vi "步骤树形列表（子VI）.vi"(5 "数据数组":string[][](array[string]), 6 "数据存储时间间隔（分钟）":dbl format="%#g", 7 "停止":bool, 8 "error out":errorcluster, 9 "queue out":refnum<queue>, 10 "数组":string[][](array[string]), 11 "notifier out":refnum<notifier>) -> (0 "当前步骤":i32, 1 "多位阀的位置":string)   [LabVIEW 2016]
uses:
  <vilib>/Utility/file.llb/Write Delimited Spreadsheet (string).vi
panel:
  out "跳转次数变量":i32=2
  out "报警器":i32
  out "电磁阀2":i32
  out "电磁阀1":i32
  out "气泵":i32
  out "蠕动泵":i32
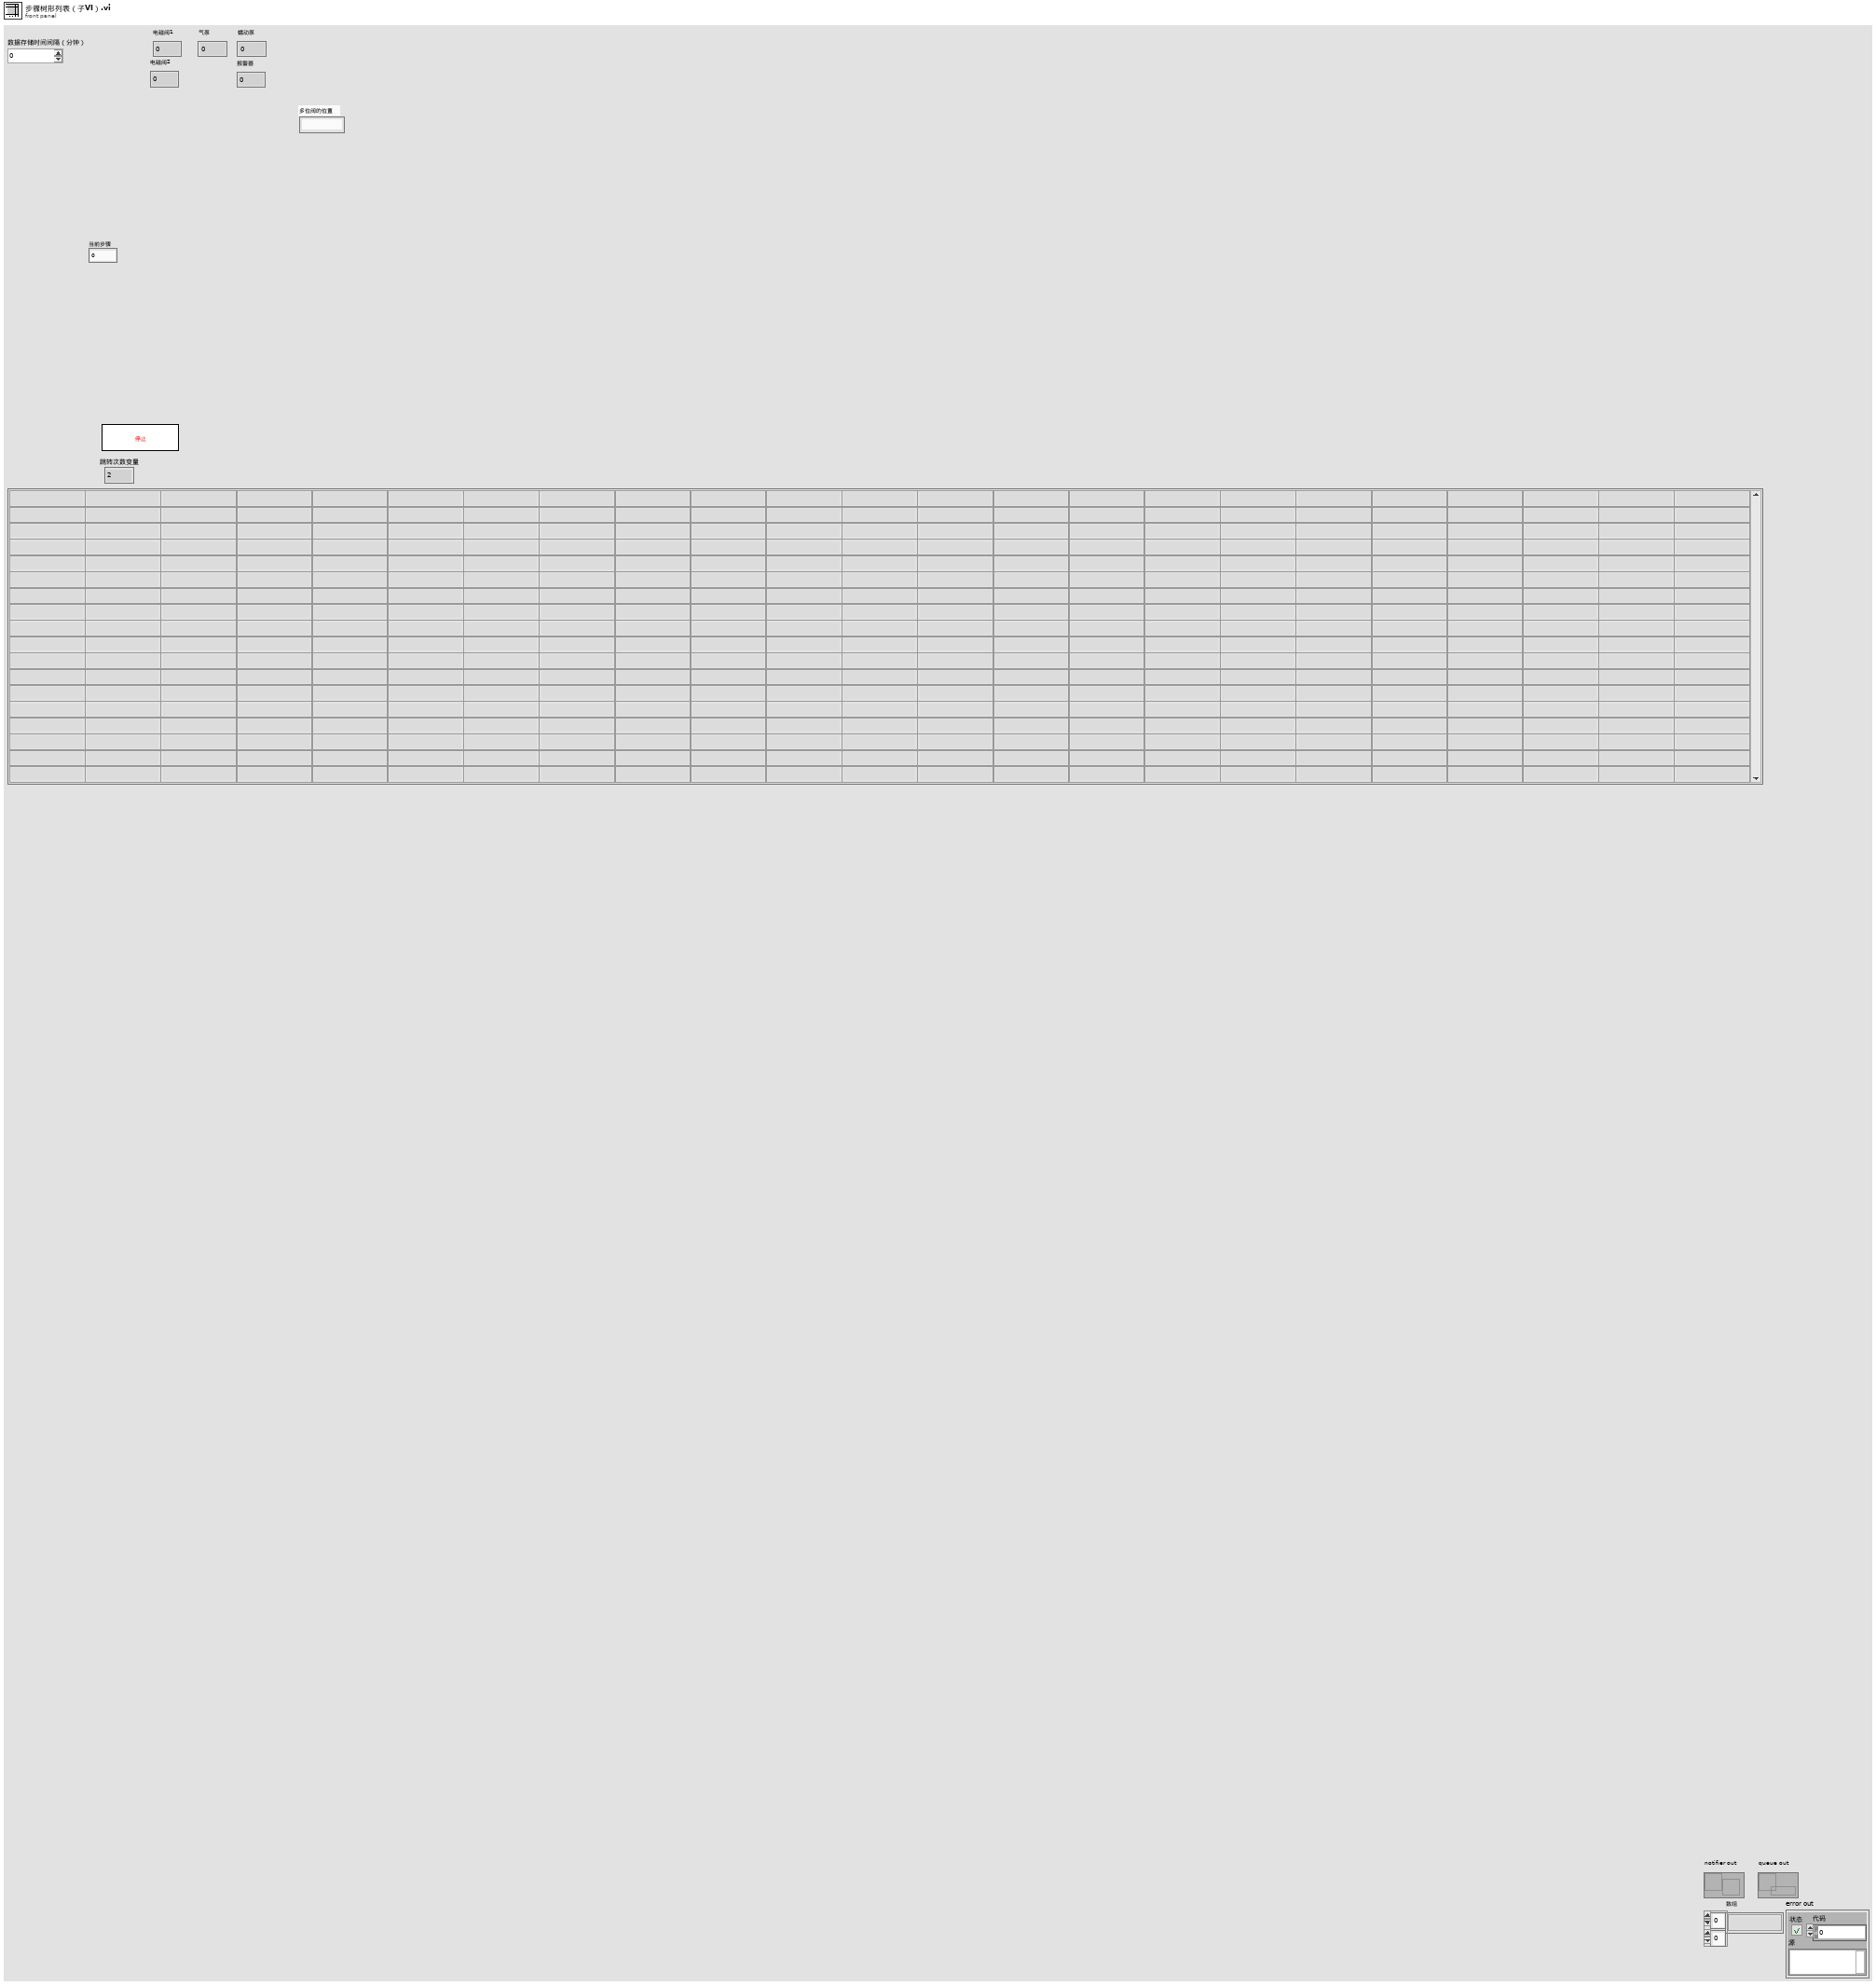
[diagram p1: front panel]
types:
  T1 = enum8{"Enabled", "Disabled", "Disabled and Grayed Out"}
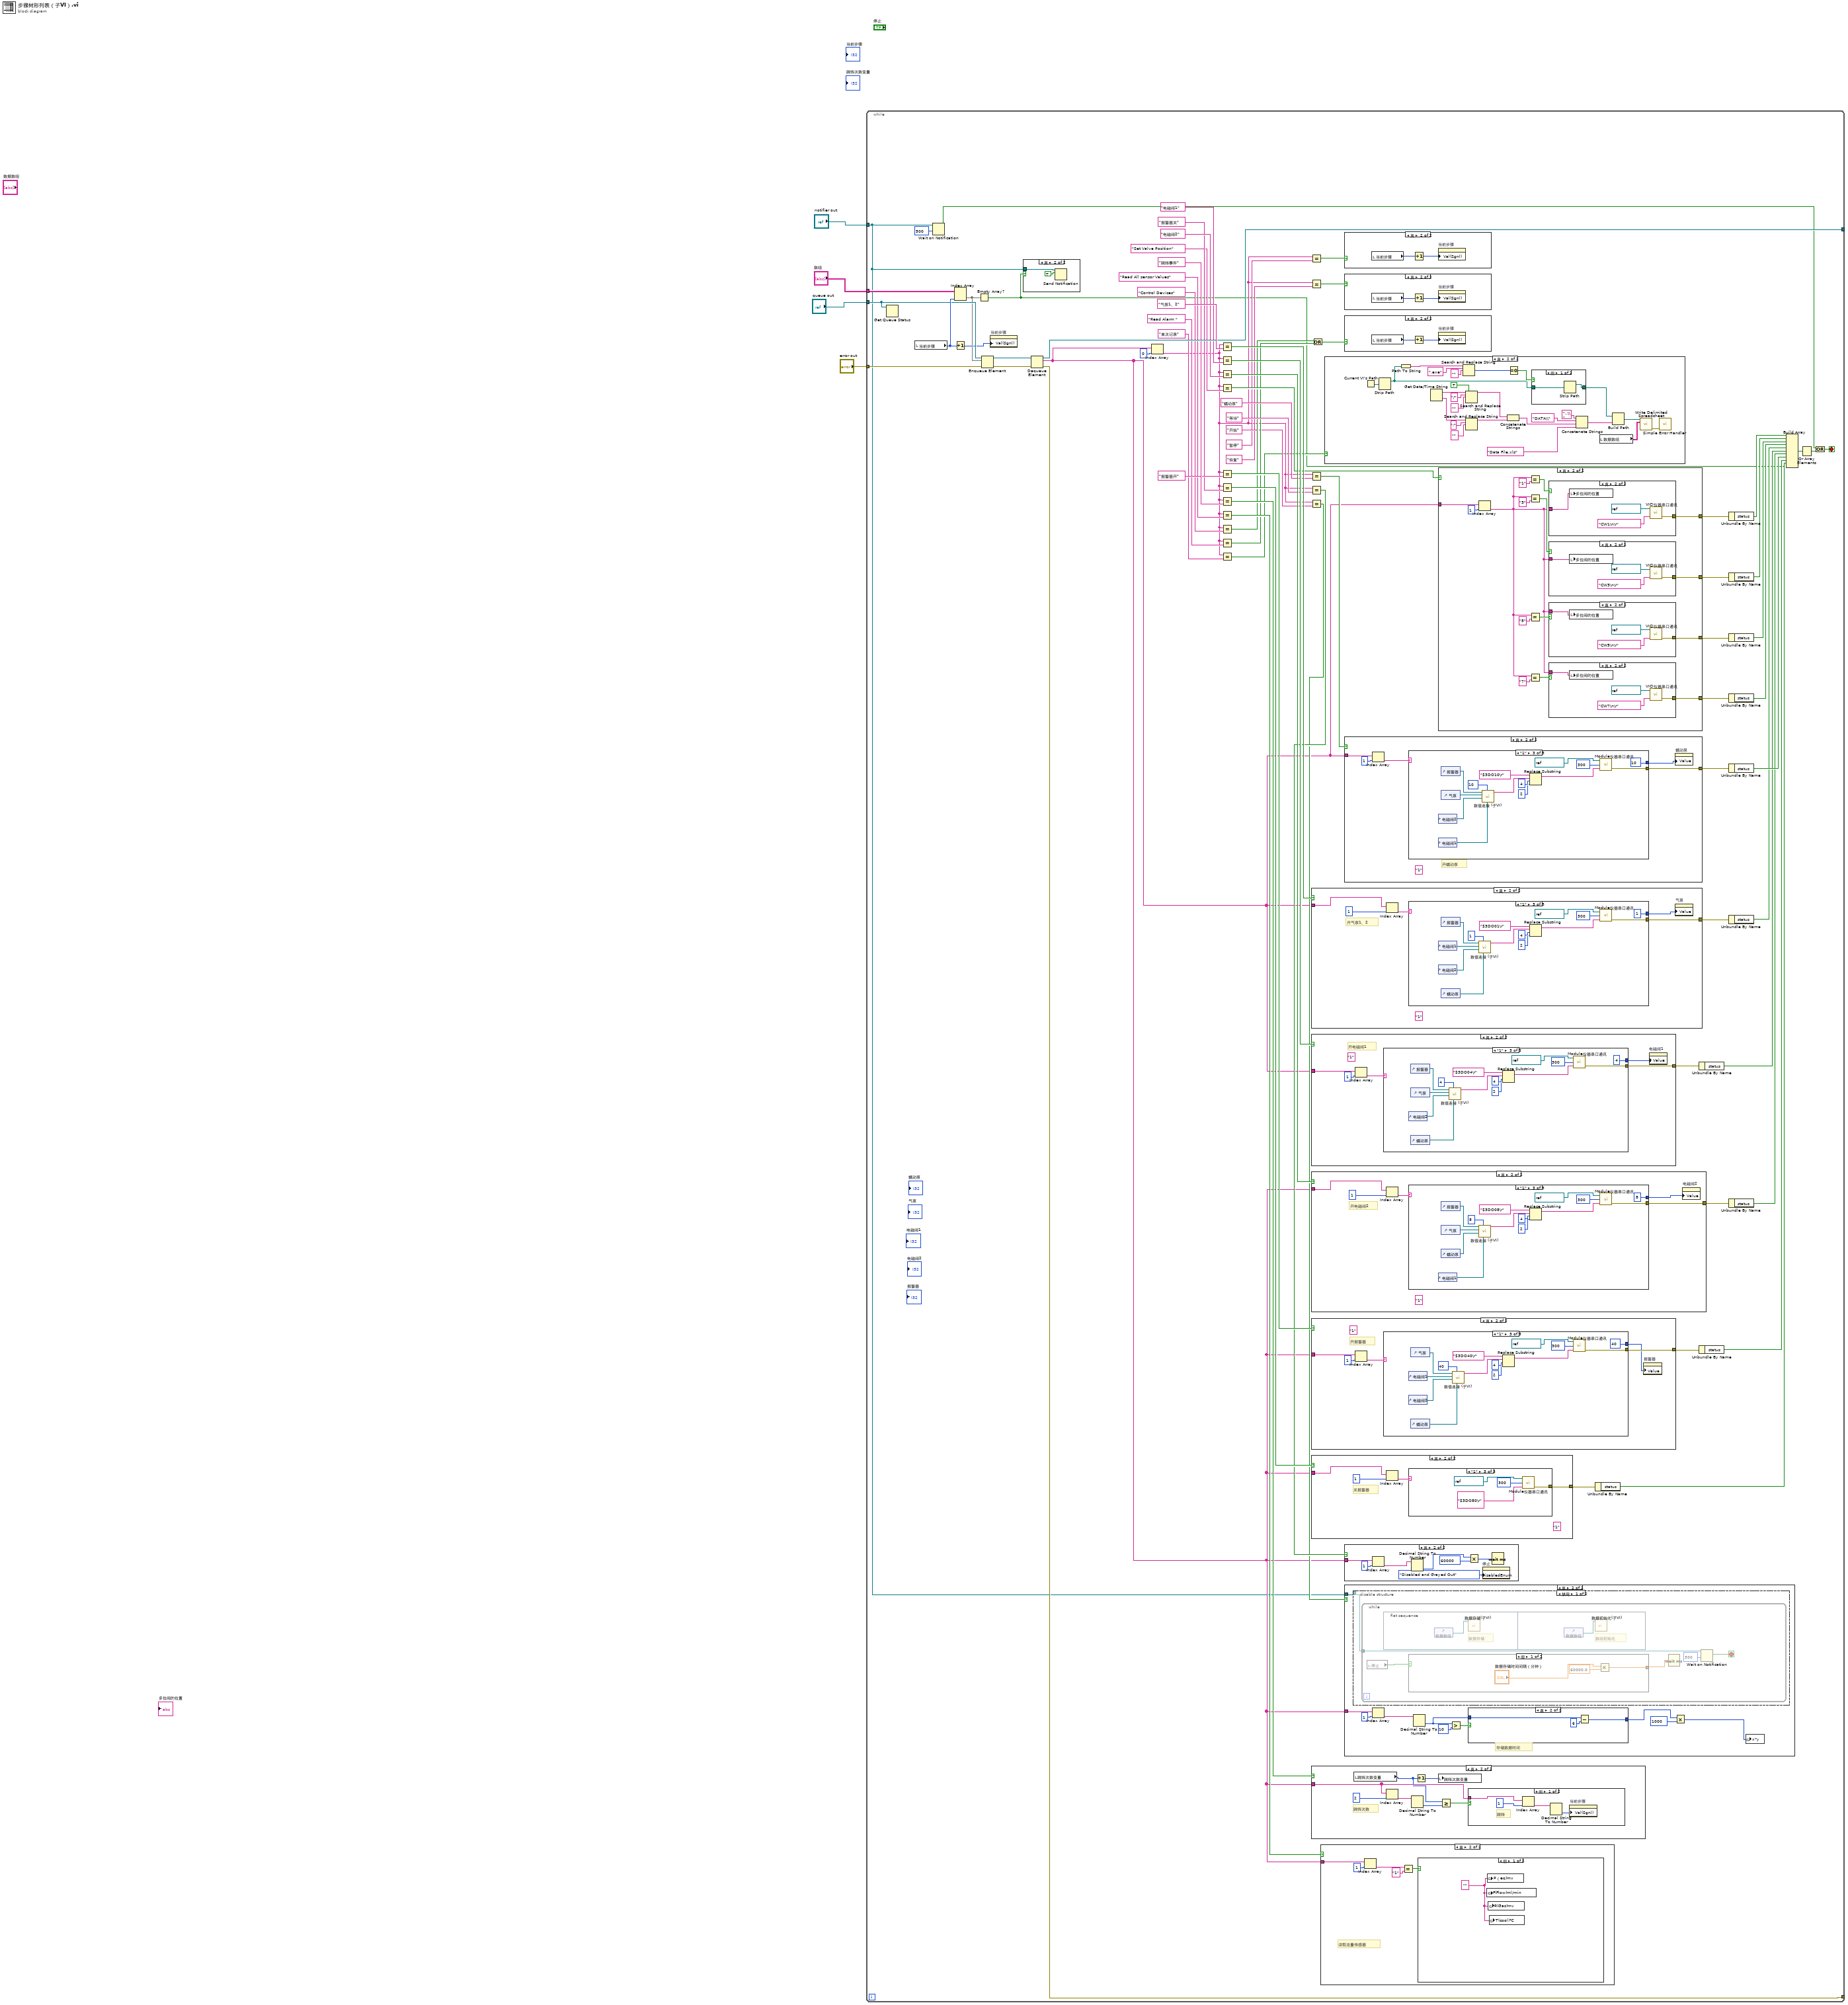
[diagram p0: block diagram]
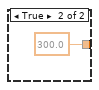
[diagram p6: hidden frame]
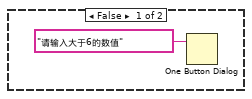
[diagram p8: hidden frame]
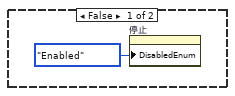
[diagram p12: hidden frame]
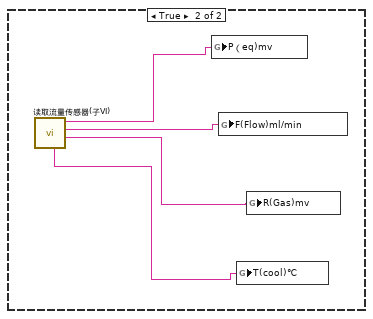
[diagram p19: hidden frame]
diagram:
  n1 = while {
    tunnel: "数组" -> [w76]
    tunnel: [w74] -> _
    tunnel: "queue out" -> [w70]
    tunnel: "error out" -> [w48]
    tunnel: [w39] -> _
    tunnel: "notifier out" -> [w5]
    stop <- w10 stop-if-true
    n2 = Get Queue Status(queue=w70) -> ()  [unwired: 2 in, 8 out]
    n3 = local read "当前步骤"() -> (w71:i32)
    n4 = Wait on Notification(notifier=w5, timeout in ms (-1)=500 ("超时毫秒(-1)")) -> (notification=w9:bool)  [unwired: 2 in, 3 out]
    n5 = Index Array(array=w76, index (col)=w71) -> (element=w69:string[])  [unwired: 1 in]
    n6 = Increment(x=w71) -> (x+1=w12:i32)
    n7 = Empty Array?(array=w69) -> (empty?=w6:bool)
    n8 = Enqueue Element(queue=w70, element=w69, error in (no error)=w48) -> (queue out=w77:refnum<queue>, error out=w49:errorcluster)  [unwired: 1 in, 1 out]
    n9 = property on="当前步骤" class="DigNum (严格)"("Val(Sgnl)"=w12) -> ()  [unwired: 2 in, 2 out]
    n10 = case shown="真" w6 {
      tunnel: w5 -> [_ w78]
      frame False {
      }
      frame True {
        n11 = Send Notification(notification=TRUE ("通知"), notifier=w78) -> ()  [unwired: 1 in, 2 out]
      }
    }
    n12 = Dequeue Element(queue=w77, error in (no error)=w49) -> (queue out=w74:refnum<queue>, element=w18:string[], error out=w39:errorcluster)  [unwired: 1 in, 1 out]
    n13 = Index Array(array=w18, index=0 ("索引")) -> (element=w15:string)
    n14 = Equal?(x=w15, y="气泵1、2") -> (x = y?=w68:bool)
    n15 = Equal?(x=w15, y="电磁阀1") -> (x = y?=w67:bool)
    n16 = Equal?(x=w15, y="电磁阀2") -> (x = y?=w64:bool)
    n17 = Equal?(x=w15, y="Set Valve Position") -> (x = y?=w55:bool)
    n18 = Equal?(x=w15, y="报警器开") -> (x = y?=w60:bool)
    n19 = Equal?(x=w15, y="报警器关") -> (x = y?=w59:bool)
    n20 = Equal?(x=w15, y="跳转事件") -> (x = y?=w72:bool)
    n21 = Equal?(x=w15, y="Read All sensor Values") -> (x = y?=w56:bool)
    n22 = Equal?(x=w15, y="Control Devices") -> (x = y?=w26:bool)
    n23 = Equal?(x=w15, y="Read Alarm ") -> (x = y?=w22:bool)
    n24 = Equal?(x=w15, y="单次记录") -> (x = y?=w7:bool)
    n25 = Equal?(x=w15, y="暂停") -> (x = y?=w14:bool)
    n26 = Equal?(x=w15, y="恢复") -> (x = y?=w13:bool)
    n27 = Equal?(x=w15, y="蠕动泵") -> (x = y?=w63:bool)
    n28 = Equal?(x=w15, y="等待") -> (x = y?=w51:bool)
    n29 = Equal?(x=w15, y="开始") -> (x = y?=w19:bool)
    n30 = case shown="真" w68 {
      tunnel: w18 -> [_ w304]
      tunnel: [_ w303] -> w50
      frame False {
      }
      frame True {
        (unwired) "1" ("y")
        # "开气泵1、2"
        n31 = Index Array(array=w304, index=1 ("索引")) -> (element=w302:string)
        n32 = case shown="\"1\"" w302 {
          tunnel: [_ w308 w323] -> w303
          tunnel: [0 0 1] -> w301
          frame "假", Default {
          }
          frame "0" {
            n33 = call "Module仪器串口通讯.vi"("输入指令"="$3DO00\r", "baud rate"=u32 300 ("baud rate (9600)"), "VISA resource name"=refnum<visa-resource-name> "COM3") -> ("错误输出"=w308:errorcluster)  [unwired: 2 out]
          }
          frame "1" {
            n34 = control-ref of="电磁阀1"() -> (w314:refnum<vi>)
            n35 = control-ref of="电磁阀2"() -> (w313:refnum<vi>)
            n36 = control-ref of="报警器"() -> (w315:refnum<vi>)
            n37 = control-ref of="蠕动泵"() -> (w312:refnum<vi>)
            n38 = call "数值连接 (子VI).vi"("DigNum引用句柄 4"=w312, "x"=1, "DigNum引用句柄 3"=w313, "DigNum引用句柄输入"=w314, "Digital输入"=w315) -> ("数据字符串"=w318:string)  [unwired: 6 in]
            n39 = Replace Substring(2:2 ("长度（子字符串长度）"), 3:4 ("偏移量(0)"), 4:w318, 5:"$3DO01\r" ("输入指令")) -> (1:w317:string)  [unwired: 1 out]
            n40 = call "Module仪器串口通讯.vi"("输入指令"=w317, "baud rate"=u32 300 ("baud rate (9600)"), "VISA resource name"=refnum<visa-resource-name> "COM3") -> ("错误输出"=w323:errorcluster)  [unwired: 2 out]
          }
        }
        n41 = property on="气泵" class="DigNum (严格)"("Value"=w301) -> ()  [unwired: 2 in, 2 out]
      }
    }
    n42 = case shown="真" w67 {
      tunnel: w18 -> [_ w279]
      tunnel: [_ w278] -> w43
      frame False {
      }
      frame True {
        (unwired) "1" ("y")
        # "开电磁阀1"
        n43 = Index Array(array=w279, index=1 ("索引")) -> (element=w277:string)
        n44 = case shown="\"1\"" w277 {
          tunnel: [_ w283 w298] -> w278
          tunnel: [0 0 4 ("电磁阀1")] -> w276
          frame "假", Default {
          }
          frame "0" {
            n45 = call "Module仪器串口通讯.vi"("输入指令"="$3DO00\r", "baud rate"=u32 300 ("baud rate (9600)"), "VISA resource name"=refnum<visa-resource-name> "COM3") -> ("错误输出"=w283:errorcluster)  [unwired: 2 out]
          }
          frame "1" {
            n46 = control-ref of="电磁阀2"() -> (w288:refnum<vi>)
            n47 = control-ref of="报警器"() -> (w290:refnum<vi>)
            n48 = control-ref of="气泵"() -> (w289:refnum<vi>)
            n49 = control-ref of="蠕动泵"() -> (w287:refnum<vi>)
            n50 = call "数值连接 (子VI).vi"("DigNum引用句柄 4"=w287, "x"=4, "DigNum引用句柄 3"=w288, "DigNum引用句柄输入"=w289, "Digital输入"=w290) -> ("数据字符串"=w295:string)  [unwired: 6 in]
            n51 = Replace Substring(2:2 ("长度（子字符串长度）"), 3:4 ("偏移量(0)"), 4:w295, 5:"$3DO04\r" ("输入指令")) -> (1:w292:string)  [unwired: 1 out]
            n52 = call "Module仪器串口通讯.vi"("输入指令"=w292, "baud rate"=u32 300 ("baud rate (9600)"), "VISA resource name"=refnum<visa-resource-name> "COM3") -> ("错误输出"=w298:errorcluster)  [unwired: 2 out]
          }
        }
        n53 = property on="电磁阀1" class="DigNum (严格)"("Value"=w276) -> ()  [unwired: 2 in, 2 out]
      }
    }
    n54 = case shown="真" w64 {
      tunnel: w18 -> [_ w254]
      tunnel: [_ w253] -> w44
      frame False {
      }
      frame True {
        (unwired) "1" ("y")
        # "开电磁阀2"
        n55 = Index Array(array=w254, index=1 ("索引")) -> (element=w252:string)
        n56 = case shown="\"1\"" w252 {
          tunnel: [_ w258 w273] -> w253
          tunnel: [0 ("电磁阀1") 0 ("电磁阀1") 8 ("电磁阀1")] -> w251
          frame "假", Default {
          }
          frame "0" {
            n57 = call "Module仪器串口通讯.vi"("输入指令"="$3DO00\r", "baud rate"=u32 300 ("baud rate (9600)"), "VISA resource name"=refnum<visa-resource-name> "COM3") -> ("错误输出"=w258:errorcluster)  [unwired: 2 out]
          }
          frame "1" {
            n58 = control-ref of="电磁阀1"() -> (w264:refnum<vi>)
            n59 = control-ref of="报警器"() -> (w262:refnum<vi>)
            n60 = control-ref of="气泵"() -> (w263:refnum<vi>)
            n61 = control-ref of="蠕动泵"() -> (w265:refnum<vi>)
            n62 = call "数值连接 (子VI).vi"("DigNum引用句柄 4"=w264, "x"=8, "DigNum引用句柄 3"=w265, "DigNum引用句柄输入"=w263, "Digital输入"=w262) -> ("数据字符串"=w270:string)  [unwired: 6 in]
            n63 = Replace Substring(2:2 ("长度（子字符串长度）"), 3:4 ("偏移量(0)"), 4:w270, 5:"$3DO08\r" ("输入指令")) -> (1:w268:string)  [unwired: 1 out]
            n64 = call "Module仪器串口通讯.vi"("输入指令"=w268, "baud rate"=u32 300 ("baud rate (9600)"), "VISA resource name"=refnum<visa-resource-name> "COM3") -> ("错误输出"=w273:errorcluster)  [unwired: 2 out]
          }
        }
        n65 = property on="电磁阀2" class="DigNum (严格)"("Value"=w251) -> ()  [unwired: 2 in, 2 out]
      }
    }
    n66 = case shown="真" w60 {
      tunnel: w18 -> [_ w204]
      tunnel: [_ w203] -> w46
      frame False {
      }
      frame True {
        (unwired) "1" ("y")
        # "开报警器"
        n67 = Index Array(array=w204, index=1 ("索引")) -> (element=w202:string)
        n68 = case shown="\"1\"" w202 {
          tunnel: [_ w208 w223] -> w203
          tunnel: [0 ("电磁阀1") 0 ("电磁阀1") 40 ("电磁阀1")] -> w201
          frame "假", Default {
          }
          frame "0" {
            n69 = call "Module仪器串口通讯.vi"("输入指令"="$3DO00\r", "baud rate"=u32 300 ("baud rate (9600)"), "VISA resource name"=refnum<visa-resource-name> "COM3") -> ("错误输出"=w208:errorcluster)  [unwired: 2 out]
          }
          frame "1" {
            n70 = control-ref of="电磁阀1"() -> (w214:refnum<vi>)
            n71 = control-ref of="电磁阀2"() -> (w213:refnum<vi>)
            n72 = control-ref of="气泵"() -> (w215:refnum<vi>)
            n73 = control-ref of="蠕动泵"() -> (w212:refnum<vi>)
            n74 = call "数值连接 (子VI).vi"("DigNum引用句柄 4"=w212, "x"=40, "DigNum引用句柄 3"=w213, "DigNum引用句柄输入"=w214, "Digital输入"=w215) -> ("数据字符串"=w221:string)  [unwired: 6 in]
            n75 = Replace Substring(2:2 ("长度（子字符串长度）"), 3:4 ("偏移量(0)"), 4:w221, 5:"$3DO40\r" ("输入指令")) -> (1:w217:string)  [unwired: 1 out]
            n76 = call "Module仪器串口通讯.vi"("输入指令"=w217, "baud rate"=u32 300 ("baud rate (9600)"), "VISA resource name"=refnum<visa-resource-name> "COM3") -> ("错误输出"=w223:errorcluster)  [unwired: 2 out]
          }
        }
        n77 = property on="报警器" class="DigNum (严格)"("Value"=w201) -> ()  [unwired: 2 in, 2 out]
      }
    }
    n78 = case shown="真" w59 {
      tunnel: w18 -> [_ w191]
      tunnel: [_ w190] -> w47
      frame False {
      }
      frame True {
        (unwired) "1" ("y")
        # "关报警器"
        n79 = Index Array(array=w191, index=1 ("索引")) -> (element=w189:string)
        n80 = case shown="\"1\"" w189 {
          tunnel: [_ w193 w197] -> w190
          frame "假", Default {
          }
          frame "0" {
            n81 = call "Module仪器串口通讯.vi"("输入指令"="$3DO00\r", "baud rate"=u32 300 ("baud rate (9600)"), "VISA resource name"=refnum<visa-resource-name> "COM3") -> ("错误输出"=w193:errorcluster)  [unwired: 2 out]
          }
          frame "1" {
            n82 = call "Module仪器串口通讯.vi"("输入指令"="$3DO80\r", "baud rate"=u32 300 ("baud rate (9600)"), "VISA resource name"=refnum<visa-resource-name> "COM3") -> ("错误输出"=w197:errorcluster)  [unwired: 2 out]
          }
        }
      }
    }
    n83 = case shown="真" w72 {
      tunnel: w18 -> [_ w327]
      frame False {
      }
      frame True {
        # "跳转次数"
        n84 = local read "跳转次数变量"() -> (w326:i32)
        n85 = Index Array(array=w327, index=2 ("索引")) -> (element=w331:string)
        n86 = Decimal String To Number(string=w331) -> (number=w328:i32)  [unwired: 2 in, 1 out]
        n87 = Increment(x=w326) -> (x+1=w330:i32)
        n88 = local write "跳转次数变量"(w330) -> ()
        n89 = Greater Or Equal?(x=w326, y=w328) -> (x >= y?=w329:bool)
        n90 = case shown="假" w329 {
          tunnel: w327 -> [w333 _]
          frame False {
            # "跳转"
            n91 = Index Array(array=w333, index=1 ("索引")) -> (element=w335:string)
            n92 = Decimal String To Number(string=w335) -> (number=w336:i32)  [unwired: 2 in, 1 out]
            n93 = property on="当前步骤" class="DigNum (严格)"("Val(Sgnl)"=w336) -> ()  [unwired: 2 in, 2 out]
          }
          frame True {
            n94 = local read "当前步骤"() -> (w338:i32)
            n95 = Increment(x=w338) -> (x+1=w337:i32)
            n96 = property on="当前步骤" class="DigNum (严格)"("Val(Sgnl)"=w337) -> ()  [unwired: 2 in, 2 out]
          }
        }
      }
    }
    n97 = Or(x=w26, y=w22) -> (x .or. y?=w25:bool)
    n98 = case shown="真" w56 {
      tunnel: w18 -> [_ w180]
      frame False {
      }
      frame True {
        # "读取流量传感器"
        n99 = Index Array(array=w180, index=1 ("索引")) -> (element=w182:string)
        n100 = Equal?(x=w182, y="1") -> (x = y?=w179:bool)
        n101 = case shown="假" w179 {
          frame False {
            w184 = "" ("T(cool)℃")
            n102 = global write "全局步骤树形列表相关.vi" "F(Flow)ml/min"(w184) -> ()
            n103 = global write "全局步骤树形列表相关.vi" "P（eq)mv"(w184) -> ()
            n104 = global write "全局步骤树形列表相关.vi" "R(Gas)mv"(w184) -> ()
            n105 = global write "全局步骤树形列表相关.vi" "T(cool)℃"(w184) -> ()
          }
          frame True {
            n106 = call "读取流量传感器(子VI).vi"() -> ("R(Gas)mv"=w186:string, "F(Flow)ml/min"=w187:string, "P（eq)mv"=w188:string, "T(cool)℃"=w185:string)  [unwired: 7 in, 1 out]
            n107 = global write "全局步骤树形列表相关.vi" "P（eq)mv"(w188) -> ()
            n108 = global write "全局步骤树形列表相关.vi" "F(Flow)ml/min"(w187) -> ()
            n109 = global write "全局步骤树形列表相关.vi" "T(cool)℃"(w185) -> ()
            n110 = global write "全局步骤树形列表相关.vi" "R(Gas)mv"(w186) -> ()
          }
        }
      }
    }
    n111 = case shown="真" w7 {
      frame False {
      }
      frame True {
        n112 = Current VI's Path() -> (path=w133:path)
        n113 = Strip Path(path=w133) -> (stripped path=w111:path)  [unwired: 1 out]
        n114 = Path To String(path=w111) -> (string=w116:string)
        n115 = Get Date/Time String() -> (date string=w127:string, time string=w130:string)  [unwired: 3 in]
        n116 = Search and Replace String(input string=w116, search string=".exe" ("搜索字符串"), replace string="" ("替换字符串(\"\")")) -> (number of replacements=w112:i32)  [unwired: 5 in, 3 out]
        n117 = Search and Replace String(replace all?=TRUE ("替换全部？(F)"), input string=w127, search string="/" ("搜索字符串"), replace string="" ("替换字符串(\"\")")) -> (result string=w123:string)  [unwired: 4 in, 3 out]
        n118 = Search and Replace String(input string=w130, search string=":" ("搜索字符串"), replace string="" ("替换字符串(\"\")")) -> (result string=w122:string)  [unwired: 5 in, 3 out]
        n119 = Concatenate Strings(w123, w122) -> (w121:string)
        n120 = Equal To 0?(x=w112) -> (x = 0?=w113:bool)
        n121 = case shown="假" w113 {
          tunnel: w111 -> [w136 w137]
          tunnel: [w135 w137] -> w110
          frame False {
            n122 = Strip Path(path=w136) -> (stripped path=w135:path)  [unwired: 1 out]
          }
          frame True {
          }
        }
        n123 = Concatenate Strings("..\\" ("字符串"), "DATA\\" ("字符串"), w121, "Data File.xls" ("name or relative path")) -> (w132:string)
        n124 = local read "数据数组"() -> (w134:string[][])
        n125 = Build Path(base path=w110, name or relative path=w132) -> (appended path=w120:path)
        n126 = call-poly <vilib>:"Write Delimited Spreadsheet.vi"("file path (dialog if empty)"=w120, "2D data"=w134) -> ("error out"=w119:errorcluster)  [unwired: 12 in, 1 out]
        n127 = call <vilib>:"Simple Error Handler.vi"("error in (no error)"=w119) -> ()  [unwired: 4 in, 5 out]
      }
    }
    n128 = case shown="真" w14 {
      frame False {
      }
      frame True {
        n129 = local read "当前步骤"() -> (w83:i32)
        n130 = Increment(x=w83) -> (x+1=w82:i32)
        n131 = property on="当前步骤" class="DigNum (严格)"("Val(Sgnl)"=w82) -> ()  [unwired: 2 in, 2 out]
      }
    }
    n132 = case shown="真" w13 {
      frame False {
      }
      frame True {
        n133 = local read "当前步骤"() -> (w81:i32)
        n134 = Increment(x=w81) -> (x+1=w80:i32)
        n135 = property on="当前步骤" class="DigNum (严格)"("Val(Sgnl)"=w80) -> ()  [unwired: 2 in, 2 out]
      }
    }
    n136 = case shown="真" w25 {
      frame False {
      }
      frame True {
        n137 = local read "当前步骤"() -> (w139:i32)
        n138 = Increment(x=w139) -> (x+1=w138:i32)
        n139 = property on="当前步骤" class="DigNum (严格)"("Val(Sgnl)"=w138) -> ()  [unwired: 2 in, 2 out]
      }
    }
    n140 = case shown="真" w63 {
      tunnel: w18 -> [_ w229]
      tunnel: [_ w228] -> w45
      frame False {
      }
      frame True {
        (unwired) "1" ("y")
        # "开蠕动泵"
        n141 = Index Array(array=w229, index=1 ("索引")) -> (element=w227:string)
        n142 = case shown="\"1\"" w227 {
          tunnel: [_ w233 w248] -> w228
          tunnel: [0 ("电磁阀1") 0 ("电磁阀1") 10 ("电磁阀1")] -> w226
          frame "假", Default {
          }
          frame "0" {
            n143 = call "Module仪器串口通讯.vi"("输入指令"="$3DO00\r", "baud rate"=u32 300 ("baud rate (9600)"), "VISA resource name"=refnum<visa-resource-name> "COM3") -> ("错误输出"=w233:errorcluster)  [unwired: 2 out]
          }
          frame "1" {
            n144 = control-ref of="电磁阀2"() -> (w240:refnum<vi>)
            n145 = control-ref of="电磁阀1"() -> (w237:refnum<vi>)
            n146 = control-ref of="报警器"() -> (w239:refnum<vi>)
            n147 = control-ref of="气泵"() -> (w238:refnum<vi>)
            n148 = call "数值连接 (子VI).vi"("DigNum引用句柄 4"=w237, "x"=10, "DigNum引用句柄 3"=w240, "DigNum引用句柄输入"=w238, "Digital输入"=w239) -> ("数据字符串"=w242:string)  [unwired: 6 in]
            n149 = Replace Substring(2:2 ("长度（子字符串长度）"), 3:4 ("偏移量(0)"), 4:w242, 5:"$3DO10\r" ("输入指令")) -> (1:w244:string)  [unwired: 1 out]
            n150 = call "Module仪器串口通讯.vi"("输入指令"=w244, "baud rate"=u32 300 ("baud rate (9600)"), "VISA resource name"=refnum<visa-resource-name> "COM3") -> ("错误输出"=w248:errorcluster)  [unwired: 2 out]
          }
        }
        n151 = property on="蠕动泵" class="DigNum (严格)"("Value"=w226) -> ()  [unwired: 2 in, 2 out]
      }
    }
    n152 = case shown="真" w51 {
      tunnel: w18 -> [_ w146]
      frame False {
        n153 = property on="停止" class="Bool (严格)"("DisabledEnum"=T1."Enabled" ("禁用")) -> ()  [unwired: 2 in, 2 out]
      }
      frame True {
        n154 = Index Array(array=w146, index=1 ("索引")) -> (element=w145:string)
        n155 = Decimal String To Number(string=w145) -> (number=w144:i32)  [unwired: 2 in, 1 out]
        n156 = Multiply(x=w144, y=60000) -> (x*y=w142:i32)
        n157 = property on="停止" class="Bool (严格)"("DisabledEnum"=T1."Disabled and Grayed Out" ("禁用")) -> ()  [unwired: 2 in, 2 out]
        n158 = Wait (ms)(milliseconds to wait=w142) -> ()  [unwired: 1 out]
      }
    }
    n159 = case shown="真" w19 {
      tunnel: w18 -> [_ w93]
      tunnel: w5 -> [_ w85]
      frame False {
      }
      frame True {
        # "存储数据时间"
        n160 = disable-structure shown="禁用" {
          disable-tunnel: w85 -> [w94 _]
          frame Disabled {
            n161 = while {
              tunnel: w94 -> [w97]
              stop <- w98 stop-if-true
              n162 = local read "停止"() -> (w99:bool)
              n163 = flat-sequence {
                frame #0 {
                  # "数据存储"
                  n164 = control-ref of="数据数组"() -> (w100:refnum<vi>)
                  n165 = call "数据存储(子VI).vi"("Array输入"=w100) -> ()  [unwired: 10 in, 1 out]
                }
                frame #1 {
                  # "数组初始化"
                  n166 = control-ref of="数据数组"() -> (w101:refnum<vi>)
                  n167 = call "数据初始化(子VI).vi"("Array输入"=w101) -> ()  [unwired: 10 in, 1 out]
                }
              }
              n168 = case shown="假" w99 {
                tunnel: [w102 300.0] -> w96
                frame False {
                  n169 = Multiply(x="数据存储时间间隔（分钟）", y=60000.0) -> (x*y=w102:dbl)
                }
                frame True {
                }
              }
              n170 = Wait (ms)(milliseconds to wait=w96) -> ()  [unwired: 1 out]
              n171 = Wait on Notification(notifier=w97, timeout in ms (-1)=300 ("超时毫秒(-1)")) -> (notification=w98:bool)  [unwired: 2 in, 3 out]
            }
          }
          frame Enabled {
          }
        }
        n172 = Index Array(array=w93, index=1 ("索引")) -> (element=w91:string)
        n173 = Decimal String To Number(string=w91) -> (number=w86:i32)  [unwired: 2 in, 1 out]
        n174 = Greater?(x=w86, y=10) -> (0:w88:bool)
        n175 = case shown="真" w88 {
          tunnel: [_ w108] -> w87
          tunnel: w86 -> [_ w109]
          frame False {
            n176 = One Button Dialog(message="请输入大于6的数值" ("消息")) -> ()  [unwired: 1 in, 1 out]
          }
          frame True {
            n177 = Subtract(x=w109, y=6) -> (x-y=w108:i32)
          }
        }
        n178 = Multiply(x=w87, y=1000) -> (x*y=w84:i32)
        n179 = global write "全局步骤树形列表相关.vi" "x*y"(w84) -> ()
      }
    }
    n180 = case shown="真" w55 {
      tunnel: w18 -> [_ w160]
      tunnel: [_ w152] -> w42
      tunnel: [_ w151] -> w41
      tunnel: [_ w150] -> w40
      tunnel: [_ w149] -> w28
      frame False {
      }
      frame True {
        n181 = Index Array(array=w160, index=1 ("索引")) -> (element=w148:string)
        n182 = Equal?(x=w148, y="1") -> (x = y?=w159:bool)
        n183 = Equal?(x=w148, y="3") -> (x = y?=w158:bool)
        n184 = Equal?(x=w148, y="5") -> (x = y?=w156:bool)
        n185 = Equal?(x=w148, y="7") -> (x = y?=w154:bool)
        n186 = case shown="真" w159 {
          tunnel: [_ w176] -> w149
          tunnel: w148 -> [_ w175]
          frame False {
          }
          frame True {
            n187 = local write "多位阀的位置"(w175) -> ()
            n188 = call "VICI仪器串口通讯.vi"("输入指令"="CW1\n\r", "VISA resource name"=refnum<visa-resource-name> "COM1") -> ("错误输出"=w176:errorcluster)  [unwired: 1 in, 2 out]
          }
        }
        n189 = case shown="真" w158 {
          tunnel: [_ w172] -> w150
          tunnel: w148 -> [_ w171]
          frame False {
          }
          frame True {
            n190 = local write "多位阀的位置"(w171) -> ()
            n191 = call "VICI仪器串口通讯.vi"("输入指令"="CW3\n\r", "VISA resource name"=refnum<visa-resource-name> "COM1") -> ("错误输出"=w172:errorcluster)  [unwired: 1 in, 2 out]
          }
        }
        n192 = case shown="真" w156 {
          tunnel: [_ w168] -> w151
          tunnel: w148 -> [_ w167]
          frame False {
          }
          frame True {
            n193 = local write "多位阀的位置"(w167) -> ()
            n194 = call "VICI仪器串口通讯.vi"("输入指令"="CW5\n\r", "VISA resource name"=refnum<visa-resource-name> "COM1") -> ("错误输出"=w168:errorcluster)  [unwired: 1 in, 2 out]
          }
        }
        n195 = case shown="真" w154 {
          tunnel: [_ w164] -> w152
          tunnel: w148 -> [_ w163]
          frame False {
          }
          frame True {
            n196 = local write "多位阀的位置"(w163) -> ()
            n197 = call "VICI仪器串口通讯.vi"("输入指令"="CW7\n\r", "VISA resource name"=refnum<visa-resource-name> "COM1") -> ("错误输出"=w164:errorcluster)  [unwired: 1 in, 2 out]
          }
        }
      }
    }
    n198 = Unbundle By Name(w47) -> ("status"=w37:bool)
    n199 = Unbundle By Name(w43) -> ("status"=w33:bool)
    n200 = Unbundle By Name(w46) -> ("status"=w38:bool)
    n201 = Unbundle By Name(w28) -> ("status"=w27:bool)
    n202 = Unbundle By Name(w40) -> ("status"=w29:bool)
    n203 = Unbundle By Name(w41) -> ("status"=w30:bool)
    n204 = Unbundle By Name(w42) -> ("status"=w31:bool)
    n205 = Unbundle By Name(w45) -> ("status"=w35:bool)
    n206 = Unbundle By Name(w50) -> ("status"=w32:bool)
    n207 = Unbundle By Name(w44) -> ("status"=w34:bool)
    n208 = Build Array(w27, w29, w30, w31, w32, w33, w34, w35, w38, w37, w6) -> (w36:bool[])
    n209 = Or Array Elements(Boolean array=w36) -> (logical OR=w11:bool)
    n210 = Or(x=w9, y=w11) -> (x .or. y?=w10:bool)
  }
